vi "ReadMessage.vi"(10 "HEX显示":bool, 11 "VISA资源名称":refnum<visa-resource-name>) -> (2 "读取缓冲区":string, 3 "VISA资源名称输出":refnum<visa-resource-name>)   [LabVIEW 2020]
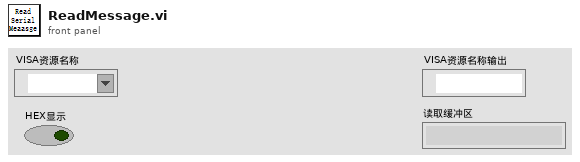
[diagram p1: front panel]
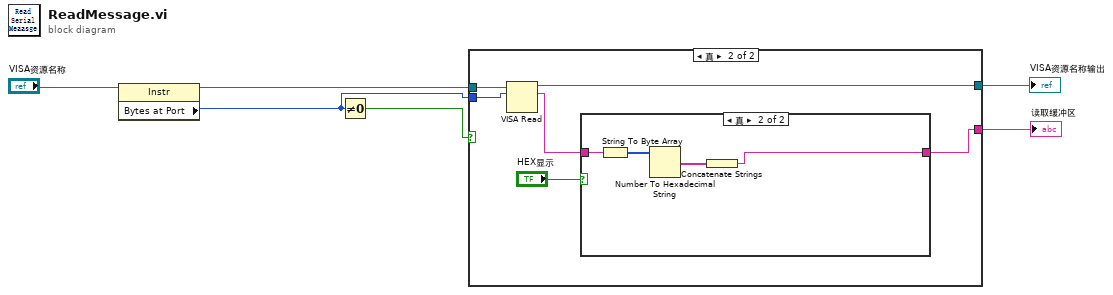
[diagram p0: block diagram]
diagram:
  n1 = property class="Instr"(reference="VISA资源名称") -> (reference out=w2:refnum<visa-resource-name>, "Bytes at Port"=w1:u32)  [unwired: 1 in, 1 out]
  n2 = Not Equal To 0?(x=w1) -> (x != 0?=w6:bool)
  n3 = case shown="真" w6 {
    tunnel: [w7 w13] -> w5
    tunnel: [_ w10] -> w4
    tunnel: w2 -> [w7 w9]
    tunnel: w1 -> [_ w8]
    frame False {
    }
    frame True {
      n4 = VISA Read(VISA resource name=w9, byte count=w8) -> (VISA resource name out=w13:refnum<visa-resource-name>, read buffer=w11:string)  [unwired: 1 in, 2 out]
      n5 = case shown="真" "HEX显示" {
        tunnel: w11 -> [w14 w18]
        tunnel: [w14 w15] -> w10
        frame False {
        }
        frame True {
          n6 = String To Byte Array(string=w18) -> (unsigned byte array=w17:u8[])
          n7 = Number To Hexadecimal String(2:w17) -> (0:w16:string[])  [unwired: 1 in]
          n8 = Concatenate Strings(w16) -> (w15:string)
        }
      }
    }
  }
  "VISA资源名称输出" <- w5
  "读取缓冲区" <- w4
